vi "Cluster-UnbundleByName.vi"() -> ()   [LabVIEW 2018]
panel:
  in  "Cluster":T1 {"Slide 2" scale=0.0..10.0; "Slide 1" scale=0.0..10.0}
  out "Gauge":dbl(knob) scale=0.0..10.0
  # "LabVIEW Cluster Demonstration"
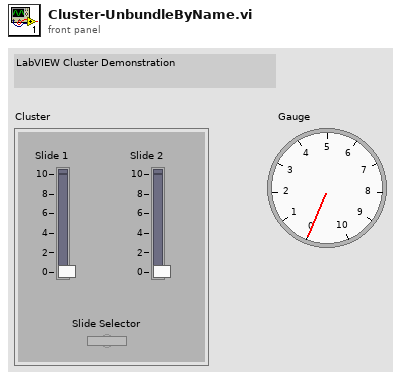
[diagram p1: front panel]
types:
  T1 = cluster{"Slide 1":dbl, "Slide 2":dbl, "Slide Selector":bool}
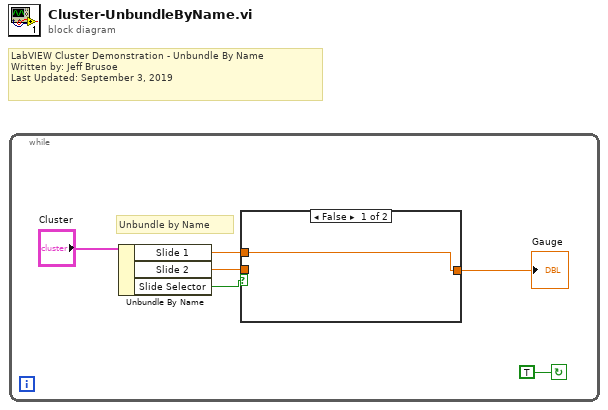
[diagram p0: block diagram]
diagram:
  # "LabVIEW Cluster Demonstration - Unbundle By Name\nWritten by: Jeff Brusoe\nLast Updated: September 3, 2019"
  n1 = while {
    stop <- TRUE continue-if-true
    # "Unbundle by Name"
    n2 = Unbundle By Name("Cluster") -> ("Slide 1"=w1:dbl, "Slide 2"=w2:dbl, "Slide Selector"=w4:bool)
    n3 = case shown="False" w4 {
      tunnel: [w7 w8] -> w3
      tunnel: w2 -> [_ w8]
      tunnel: w1 -> [w7 _]
      frame False {
      }
      frame True {
      }
    }
    "Gauge" <- w3
  }
